vi "nD Line Search (VI).vi"(5 "J":dbl[][](array[numeric]) format="%.2f", 6 "data":variant, 7 "F(X)":T1, 8 "TOLX":dbl=1e-07 format="%.2e", 9 "alpha":dbl=0.0001 format="%.2e", 10 "P":dbl[](array[numeric]) format="%.2f", 11 "X":dbl[](array[numeric]) format="%.2f") -> (0 "error":i32, 2 "index":u32, 3 "X (new)":dbl[](array[numeric]) format="%.2f")   [LabVIEW 2020, in "NI_Gmath.lvlib"]
uses:
  NI_Gmath.lvlib
  functionRefnum nD.ctl
  NI_AALBase.lvlib
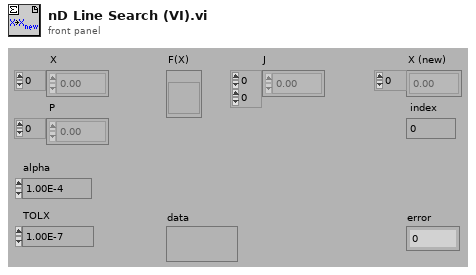
[diagram p1: front panel]
types:
  T1 = typedef "NI_Gmath.lvlib/functionRefnum nD.ctl" = refnum<vi>
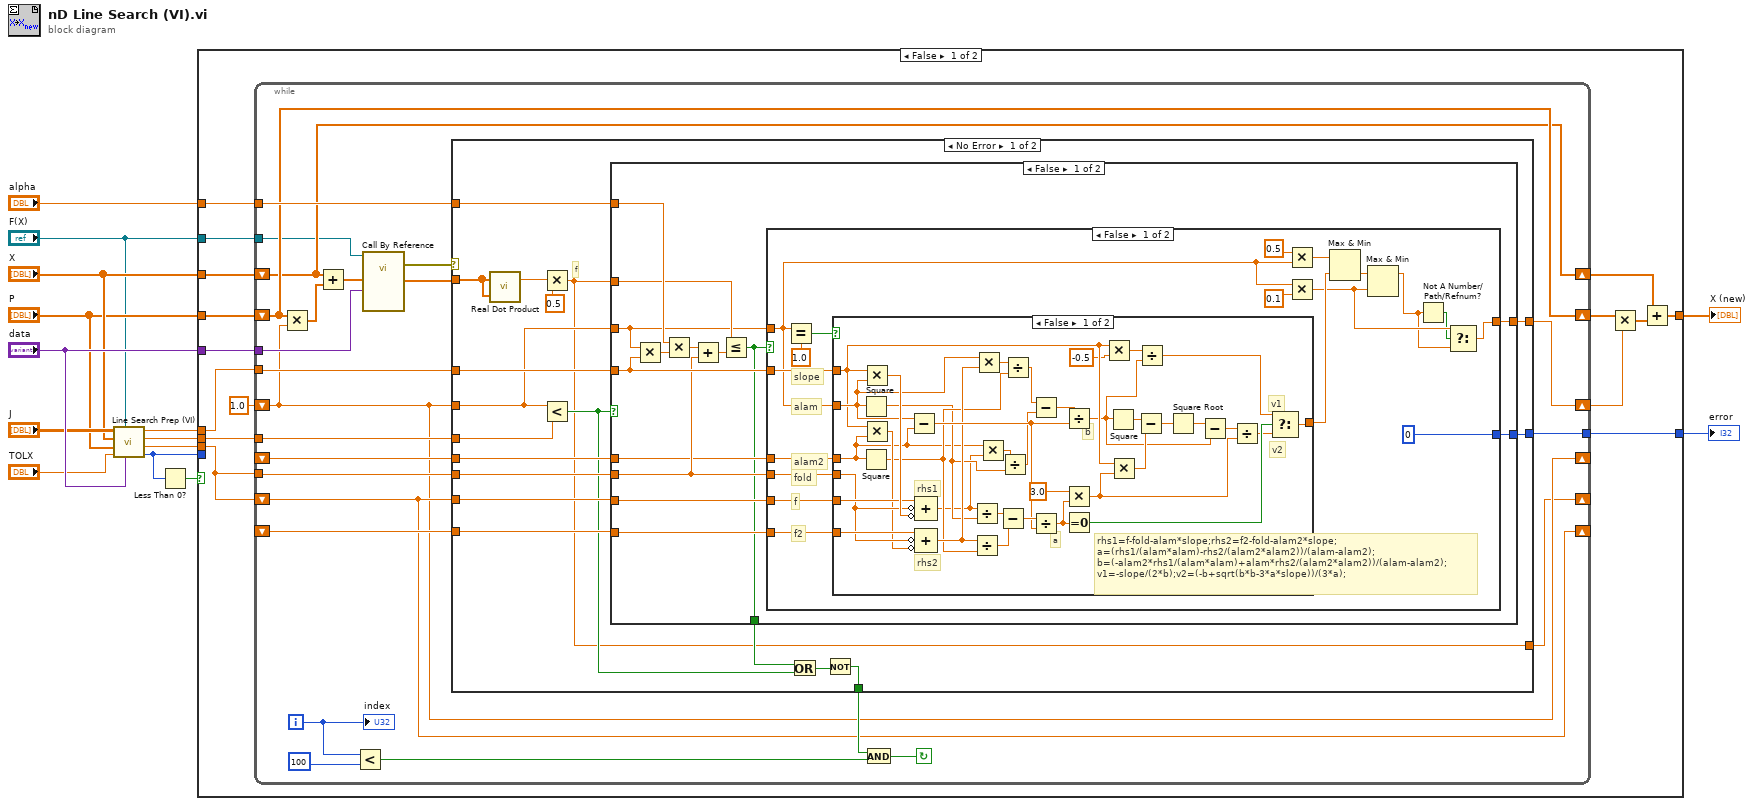
[diagram p0: block diagram]
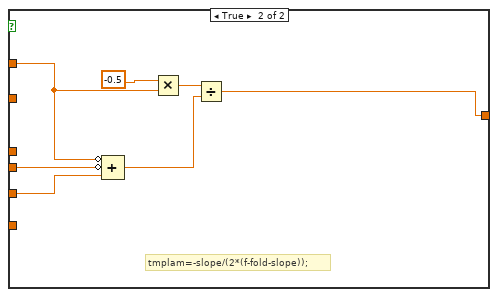
[diagram p2: hidden frame]
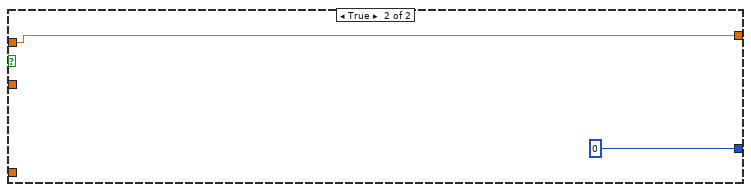
[diagram p3: hidden frame]
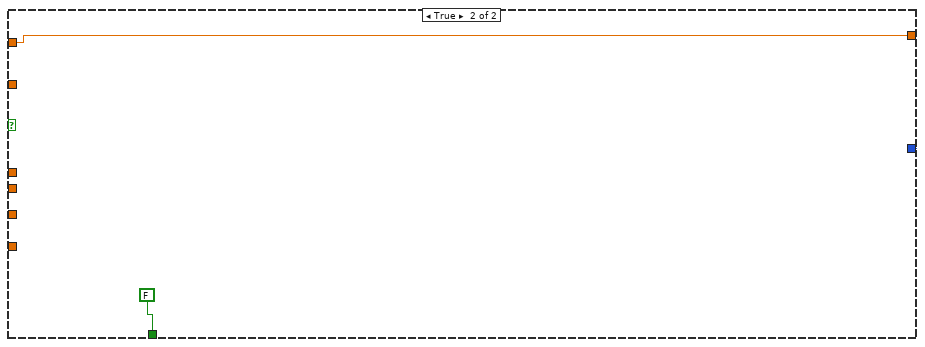
[diagram p4: hidden frame]
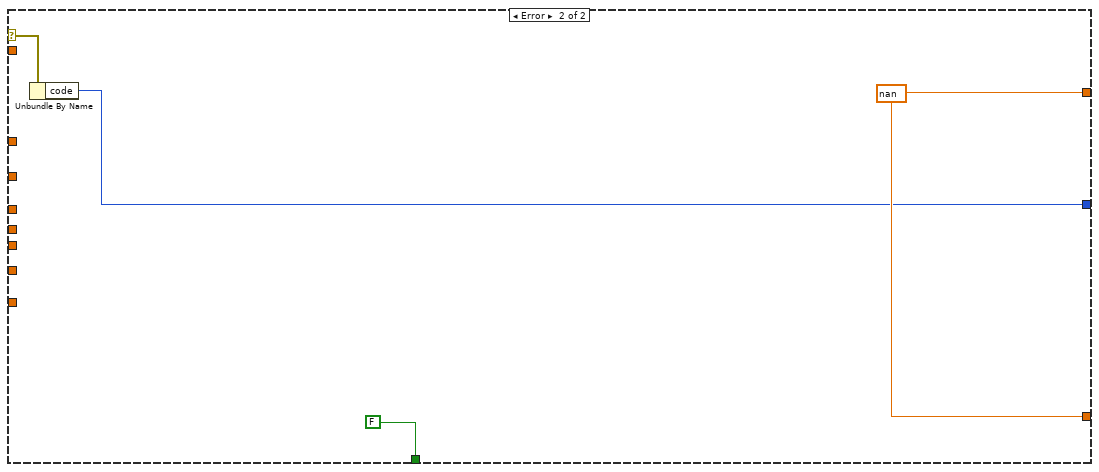
[diagram p5: hidden frame]
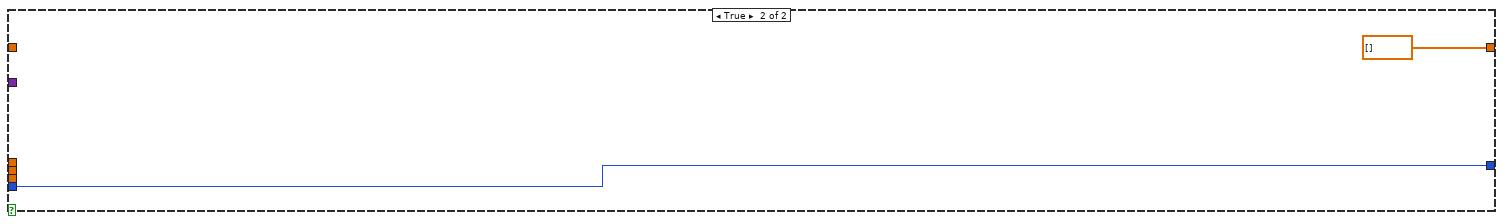
[diagram p6: hidden frame]
diagram:
  n1 = call "Line Search Prep (VI).vi"("data"="data", "F(X)"="F(X)", "TOLX"="TOLX", "P"="P", "X"="X", "J"="J") -> ("error"=w3:i32, "F(X)*F(X)"=w9:dbl, "tolerance"=w11:dbl, "X * Y"=w10:dbl)  [unwired: 2 out]
  n2 = Less Than 0?(x=w3) -> (x < 0?=w4:bool)
  n3 = case shown="False" w4 {
    tunnel: "data" -> [w29 _]
    tunnel: w11 -> [w27 _]
    tunnel: w10 -> [w26 _]
    tunnel: w9 -> [w25 _]
    tunnel: [w20 dbl[] []] -> w8
    tunnel: "alpha" -> [w19 _]
    tunnel: "X" -> [w18 _]
    tunnel: "P" -> [w17 _]
    tunnel: "F(X)" -> [w16 _]
    tunnel: w3 -> [_ w157]
    tunnel: [w15 w157] -> w2
    frame False {
      n4 = while {
        tunnel: w25 -> [w49]
        tunnel: w26 -> [w50]
        tunnel: w19 -> [w51]
        tunnel: w27 -> [w52]
        shift-left: _ -> [w48]
        shift-right: [w35] -> _
        shift-left: w25 -> [w35]
        shift-right: [w32] -> _
        shift-left: _ -> [w47]
        shift-right: [w34] -> _
        shift-left: 1.0 -> [w34]
        shift-right: [w43] -> w23
        shift-left: w17 -> [w46]
        shift-right: [w46] -> w22
        shift-left: w18 -> [w45]
        shift-right: [w45] -> w24
        tunnel: w16 -> [w38]
        tunnel: w29 -> [w37]
        tunnel: [w33] -> w15
        i -> [w44]
        stop <- w39 continue-if-true
        n5 = Multiply(x=w46, y=w34) -> (x*y=w53:dbl[])
        n6 = Add(x=w45, y=w53) -> (x+y=w31:dbl[])
        n7 = Less?(x=w44, y=100) -> (x < y?=w41:bool)
        n8 = call-by-ref "?"(reference=w38, "variant"=w37, "X"=w31) -> (error out=w30:errorcluster, "F(X)"=w36:dbl[])  [unwired: 4 in, 1 out]
        n9 = case shown="No Error" w30 {
          selector: w30 -> [_ w153]
          tunnel: w52 -> [w71 _]
          tunnel: w51 -> [w70 _]
          tunnel: w50 -> [w69 _]
          tunnel: w49 -> [w68 _]
          tunnel: w35 -> [w64 _]
          tunnel: w48 -> [w63 _]
          tunnel: w47 -> [w62 _]
          tunnel: [w59 w154] -> w43
          tunnel: [w58 FALSE] -> w40
          tunnel: w36 -> [w57 _]
          tunnel: w34 -> [w56 _]
          tunnel: [w55 w154] -> w32
          tunnel: [w54 w152] -> w33
          frame No Error {
            # "f"
            n10 = call "Real Dot Product.vi"("Y Vector"=w57, "X Vector"=w57) -> ("X * Y"=w67:dbl)  [unwired: 1 out]
            n11 = Multiply(x=w67, y=0.5) -> (x*y=w55:dbl)
            n12 = Less?(x=w56, y=w71) -> (x < y?=w61:bool)
            n13 = case shown="False" w61 {
              tunnel: w70 -> [w85 _]
              tunnel: w56 -> [w80 w150]
              tunnel: w69 -> [w78 _]
              tunnel: w68 -> [w76 _]
              tunnel: w55 -> [w81 _]
              tunnel: [w73 FALSE] -> w65
              tunnel: [w79 w150] -> w59
              tunnel: w64 -> [w77 _]
              tunnel: w63 -> [w75 _]
              tunnel: w62 -> [w74 _]
              tunnel: [w72 0] -> w54
              frame False {
                n14 = Multiply(x=w80, y=w78) -> (x*y=w84:dbl)
                n15 = Multiply(x=w85, y=w84) -> (x*y=w83:dbl)
                n16 = Add(x=w83, y=w76) -> (x+y=w82:dbl)
                n17 = Less Or Equal?(x=w81, y=w82) -> (x <= y?=w73:bool)
                n18 = case shown="False" w73 {
                  tunnel: w80 -> [w93 w148]
                  tunnel: [w87 w148] -> w79
                  tunnel: w78 -> [w96 _]
                  tunnel: w77 -> [w95 _]
                  tunnel: w76 -> [w94 _]
                  tunnel: w75 -> [w92 _]
                  tunnel: w74 -> [w91 _]
                  tunnel: [0 0] -> w72
                  frame False {
                    # "f2"
                    # "f"
                    # "slope"
                    # "fold"
                    # "alam2"
                    # "alam"
                    n19 = Equal?(x=w93, y=1.0) -> (x = y?=w102:bool)
                    n20 = case shown="False" w102 {
                      tunnel: [w138 w140] -> w99
                      tunnel: w96 -> [w108 w141]
                      tunnel: w95 -> [w136 w146]
                      tunnel: w94 -> [w134 w145]
                      tunnel: w93 -> [w119 _]
                      tunnel: w92 -> [w135 _]
                      tunnel: w91 -> [w112 _]
                      frame False {
                        # "rhs1=f-fold-alam*slope;rhs2=f2-fold-alam2*slope;\na=(rhs1/(alam*alam)-rhs2/(alam2*alam2))/(alam-alam2);\nb=(-alam2*rhs1/(alam*alam)+alam*rhs2/(alam2*alam2))/(alam-alam2);\nv1=-slope/(2*b);v2=(-b+sqrt(b*b-3*a*slope))/(3*a);"
                        # "rhs2"
                        # "rhs1"
                        # "b"
                        # "v2"
                        # "v1"
                        # "a"
                        n21 = Square(x=w119) -> (x^2=w113:dbl)
                        n22 = Square(x=w112) -> (x^2=w116:dbl)
                        n23 = Multiply(x=w108, y=w119) -> (x*y=w137:dbl)
                        n24 = Multiply(x=w108, y=w112) -> (x*y=w133:dbl)
                        n25 = Subtract(x=w119, y=w112) -> (x-y=w129:dbl)
                        n26 = Compound Arithmetic op=ADD(w136, invert w134, invert w137) -> (w111:dbl)
                        n27 = Compound Arithmetic op=ADD(w135, invert w134, invert w133) -> (w118:dbl)
                        n28 = Divide(x=w111, y=w113) -> (x/y=w114:dbl)
                        n29 = Divide(x=w118, y=w116) -> (x/y=w132:dbl)
                        n30 = Multiply(x=w119, y=w118) -> (x*y=w117:dbl)
                        n31 = Multiply(x=w112, y=w111) -> (x*y=w110:dbl)
                        n32 = Subtract(x=w114, y=w132) -> (x-y=w131:dbl)
                        n33 = Divide(x=w110, y=w113) -> (x/y=w109:dbl)
                        n34 = Divide(x=w117, y=w116) -> (x/y=w115:dbl)
                        n35 = Subtract(x=w115, y=w109) -> (x-y=w130:dbl)
                        n36 = Divide(x=w131, y=w129) -> (x/y=w124:dbl)
                        n37 = Divide(x=w130, y=w129) -> (x/y=w105:dbl)
                        n38 = Multiply(x=3.0, y=w124) -> (x*y=w121:dbl)
                        n39 = Equal To 0?(x=w124) -> (x = 0?=w139:bool)
                        n40 = Multiply(x=w108, y=-0.5) -> (x*y=w106:dbl)
                        n41 = Square(x=w105) -> (x^2=w128:dbl)
                        n42 = Multiply(x=w108, y=w121) -> (x*y=w123:dbl)
                        n43 = Subtract(x=w128, y=w123) -> (x-y=w127:dbl)
                        n44 = Divide(x=w106, y=w105) -> (x/y=w104:dbl)
                        n45 = Square Root(x=w127) -> (sqrt(x)=w126:dbl)
                        n46 = Subtract(x=w126, y=w105) -> (x-y=w122:dbl)
                        n47 = Divide(x=w122, y=w121) -> (x/y=w120:dbl)
                        n48 = Select(t=w104, s=w139, f=w120) -> (s? t:f=w138:dbl)
                      }
                      frame True {
                        # "tmplam=-slope/(2*(f-fold-slope));"
                        n49 = Compound Arithmetic op=ADD(invert w141, invert w145, w146) -> (w143:dbl)
                        n50 = Multiply(x=-0.5, y=w141) -> (x*y=w144:dbl)
                        n51 = Divide(x=w144, y=w143) -> (x/y=w140:dbl)
                      }
                    }
                    n52 = Multiply(x=0.5, y=w93) -> (x*y=w100:dbl)
                    n53 = Multiply(x=w93, y=0.1) -> (x*y=w89:dbl)
                    n54 = Max & Min(x=w100, y=w99) -> (min(x,y)=w97:dbl)  [unwired: 1 out]
                    n55 = Max & Min(x=w97, y=w89) -> (max(x,y)=w88:dbl)  [unwired: 1 out]
                    n56 = Not A Number/Path/Refnum?(number/path/refnum=w88) -> (NaN/Path/Refnum?=w86:bool)
                    n57 = Select(t=w89, s=w86, f=w88) -> (s? t:f=w87:dbl)
                  }
                  frame True {
                  }
                }
              }
              frame True {
              }
            }
            n58 = Or(x=w65, y=w61) -> (x .or. y?=w60:bool)
            n59 = Not(x=w60) -> (.not. x?=w58:bool)
          }
          frame Error {
            w154 = nan
            n60 = Unbundle By Name(w153) -> ("code"=w152:i32)
          }
        }
        n61 = And(x=w40, y=w41) -> (x .and. y?=w39:bool)
        "index" <- w44
      }
      n62 = Multiply(x=w22, y=w23) -> (x*y=w21:dbl[])
      n63 = Add(x=w24, y=w21) -> (x+y=w20:dbl[])
    }
    frame True {
    }
  }
  "X (new)" <- w8
  "error" <- w2
